vi "changeState.vi"(8 "error in (no error)":errorcluster, 10 "State":u16, 11 "Subnet in":refnum<class "Subnet.lvclass">) -> (0 "error out":errorcluster, 3 "Subnet out":refnum<class "Subnet.lvclass">)   [LabVIEW 2016, in "Subnet.lvclass"]
uses:
  Subnet.lvclass
  Subnet.lvclass/Subnet.ctl
  Common_RT_ILC/ILC/ILC.lvclass/ILC.ctl
  Common_RT_HPILC/HPILC/HPILC.lvclass
  D:/Code/Common_RT_ILC/ILC/ILC.lvclass
  Common_RT_MTILC/MTILC/MTILC.lvclass
  Common_RT_MDILC/MDILC/MDILC.lvclass
  Common_RT_MIILC/MIILC/MIILC.lvclass
  Common_RT_Modbus/IModbus/IModbus.lvclass
  Common_RT_ILC/ILC/ILC.lvclass
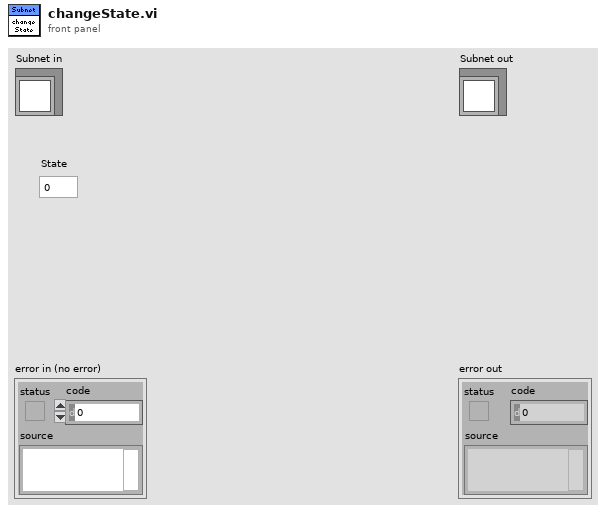
[diagram p1: front panel]
types:
  T1 = typedef "RTILC.lvlib/ILCData.ctl" = cluster{"Constants":T2, "Command":T3, "Telemetry":T5, "Responses":T6, "Timings":T8}
  T2 = typedef "RTILC.lvlib/ILCConstants.ctl" = cluster{"Subnet":u8, "Address":u8}
  T3 = typedef "RTILC.lvlib/ILCCommand.ctl" = cluster{"ILCMode":u16, "TemporaryAddress":u8, "ADCScanRate":T4, "ADCChannel":u8, "ADCOffset":sgl, "ADCSensitivity":sgl}
  T4 = typedef "RTILC.lvlib/ILCScanRates.ctl" = u8
  T5 = typedef "RTILC.lvlib/ILCTelemetry.ctl" = cluster{"UniqueID":u64, "FirmwareType":u8, "NetworkNodeType":u8, "ILCOption":u8, "NetworkNodeOption":u8, "MajorRevision":u8, "MinorRevision":u8, "FirmwareName":string, "ILCMode":u16, "MajorFault":bool, "MinorFault":bool, "FaultOverride":bool, "UniqueIDCRCMismatch":bool, "AppTypeNodeTypeMismatch":bool, "AppMissing":bool, "AppCRCMismatch":bool, "TEDSNotFound":bool, "TEDS1Mismatch":bool, "TEDS2Mismatch":bool, "WatchdogResetDetected":bool, "BrownoutDetected":bool, "EventTrapResetDetected":bool, "TemporaryAddress":u8, "ADCScanRate":T4, "DAC1":u16, "DAC2":u16, "DAC3":u16, "DAC4":u16, "MainADCCalibrationK":sgl[], "MainSensorOffset":sgl[], "MainSensorSensitivity":sgl[], "BackupADCCalibrationK":sgl[], "BackupSensorOffset":sgl[], "BackupSensorSensitivity":sgl[]}
  T6 = typedef "RTILC.lvlib/ILCResponses.ctl" = cluster{"ReportServerID":T7, "ReportServerStatus":T7, "ILCMode":T7, "SetTemporaryAddress":T7, "Reset":T7, "ADCScanRate":T7, "ADCOffsetSensitivity":T7, "ReadDAC":T7, "ReadCalibration":T7}
  T7 = typedef "RTModbus.lvlib/ExceptionCodes.ctl" = u16
  T8 = typedef "RTILC.lvlib/ILCTimings.ctl" = cluster{"ADCOffsetSensitivity":u32, "ADCScanRate":u32, "ILCMode":u32, "ReadCalibration":u32, "ReportServerID":u32, "ReportServerStatus":u32, "Reset":u32, "SetTemporaryAddress":u32}
  T9 = typedef "RTModbus.lvlib/TxFrame.ctl" = cluster{"Data":u8[], "WaitForTrigger":bool, "WaitForRx":u16, "TriggerIRQ":bool, "DelayMicroseconds":u16, "DelayMilliseconds":u16, "Timestamp":bool}
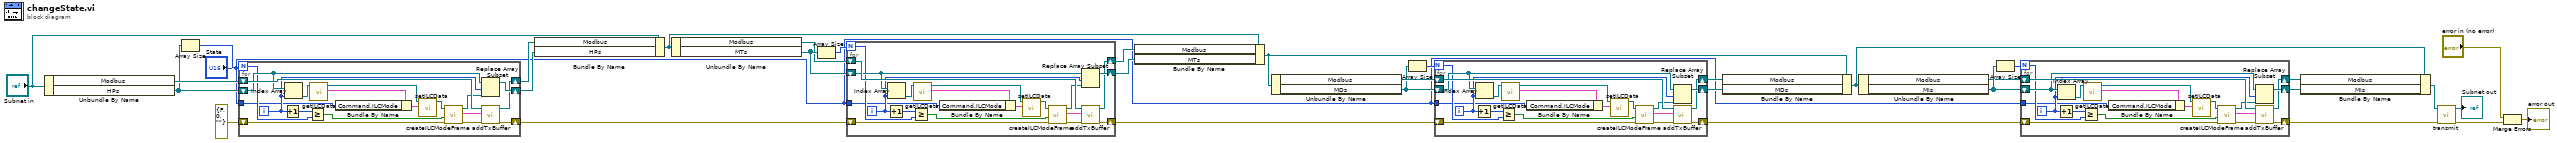
[diagram p0: block diagram]
diagram:
  n1 = Unbundle By Name("Subnet in") -> ("Modbus"=w35:refnum<class "IModbus.lvclass">, "HPs"=w34:refnum<class "HPILC.lvclass">[])
  n2 = Array Size(array=w34) -> (size(s)=w33:i32)
  n3 = for {
    N: w33 -> [w38]
    shift-right: [w44] -> w31
    shift-left: w35 -> [w49]
    shift-right: [w45] -> w30
    shift-left: w34 -> [w47]
    shift-right: [w42] -> w4
    shift-left: errorcluster {"status"=FALSE, "code"=0, "source"=""} ("error out") -> [w41]
    tunnel: "State" -> [w36]
    i -> [w40]
    n4 = Increment(x=w40) -> (x+1=w39:i32)
    n5 = Index Array(array=w47, index=w40) -> (element=w48:refnum<class "HPILC.lvclass">)
    n6 = Greater Or Equal?(x=w39, y=w38) -> (x >= y?=w37:bool)
    n7 = call "getILCData.vi"("ILC in"=w48) -> ("ILCData"=w53:T1, "ILC out"=w54:refnum<class "HPILC.lvclass">)  [unwired: 9 in]
    n8 = Bundle By Name(cluster=w53, "Command.ILCMode"=w36) -> (w52:T1)
    n9 = call "setILCData.vi"("ILCData"=w52, "ILC in"=w54) -> ("ILC out"=w51:refnum<class "HPILC.lvclass">)  [unwired: 9 in]
    n10 = call "createILCModeFrame.vi"("error in (no error)"=w41, "TriggerIRQ"=w37, "ILC in"=w51) -> ("error out"=w43:errorcluster, "TxFrame"=w50:T9, "ILC out"=w46:refnum<class "HPILC.lvclass">)  [unwired: 6 in]
    n11 = Replace Array Subset(array=w47, new element=w46, index=w40) -> (w45:refnum<class "HPILC.lvclass">[])
    n12 = call-dynamic "addTxBuffer.vi"("error in (no error)"=w43, "TxFrame"=w50, "IModbus in"=w49) -> ("error out"=w42:errorcluster, "IModbus out"=w44:refnum<class "IModbus.lvclass">)  [unwired: 7 in]
  }
  n13 = Bundle By Name(cluster="Subnet in", "Modbus"=w31, "HPs"=w30) -> (w19:refnum<class "Subnet.lvclass">)
  n14 = Unbundle By Name(w19) -> ("Modbus"=w20:refnum<class "IModbus.lvclass">, "MTs"=w21:refnum<class "MTILC.lvclass">[])
  n15 = Array Size(array=w21) -> (size(s)=w22:i32)
  n16 = for {
    N: w22 -> [w57]
    shift-right: [w63] -> w23
    shift-left: w20 -> [w68]
    shift-right: [w64] -> w24
    shift-left: w21 -> [w66]
    shift-right: [w61] -> w5
    shift-left: w4 -> [w60]
    tunnel: "State" -> [w55]
    i -> [w59]
    n17 = Increment(x=w59) -> (x+1=w58:i32)
    n18 = Index Array(array=w66, index=w59) -> (element=w67:refnum<class "MTILC.lvclass">)
    n19 = Greater Or Equal?(x=w58, y=w57) -> (x >= y?=w56:bool)
    n20 = call "getILCData.vi"("ILC in"=w67) -> ("ILCData"=w72:T1, "ILC out"=w73:refnum<class "MTILC.lvclass">)  [unwired: 9 in]
    n21 = Bundle By Name(cluster=w72, "Command.ILCMode"=w55) -> (w71:T1)
    n22 = call "setILCData.vi"("ILCData"=w71, "ILC in"=w73) -> ("ILC out"=w70:refnum<class "MTILC.lvclass">)  [unwired: 9 in]
    n23 = call "createILCModeFrame.vi"("error in (no error)"=w60, "TriggerIRQ"=w56, "ILC in"=w70) -> ("error out"=w62:errorcluster, "TxFrame"=w69:T9, "ILC out"=w65:refnum<class "MTILC.lvclass">)  [unwired: 6 in]
    n24 = Replace Array Subset(array=w66, new element=w65, index=w59) -> (w64:refnum<class "MTILC.lvclass">[])
    n25 = call-dynamic "addTxBuffer.vi"("error in (no error)"=w62, "TxFrame"=w69, "IModbus in"=w68) -> ("error out"=w61:errorcluster, "IModbus out"=w63:refnum<class "IModbus.lvclass">)  [unwired: 7 in]
  }
  n26 = Bundle By Name(cluster=w19, "Modbus"=w23, "MTs"=w24) -> (w13:refnum<class "Subnet.lvclass">)
  n27 = Unbundle By Name(w13) -> ("Modbus"=w18:refnum<class "IModbus.lvclass">, "MDs"=w17:refnum<class "MDILC.lvclass">[])
  n28 = Array Size(array=w17) -> (size(s)=w16:i32)
  n29 = for {
    N: w16 -> [w76]
    shift-right: [w82] -> w15
    shift-left: w18 -> [w87]
    shift-right: [w83] -> w14
    shift-left: w17 -> [w85]
    shift-right: [w80] -> w6
    shift-left: w5 -> [w79]
    tunnel: "State" -> [w74]
    i -> [w78]
    n30 = Increment(x=w78) -> (x+1=w77:i32)
    n31 = Index Array(array=w85, index=w78) -> (element=w86:refnum<class "MDILC.lvclass">)
    n32 = Greater Or Equal?(x=w77, y=w76) -> (x >= y?=w75:bool)
    n33 = call "getILCData.vi"("ILC in"=w86) -> ("ILCData"=w91:T1, "ILC out"=w92:refnum<class "MDILC.lvclass">)  [unwired: 9 in]
    n34 = Bundle By Name(cluster=w91, "Command.ILCMode"=w74) -> (w90:T1)
    n35 = call "setILCData.vi"("ILCData"=w90, "ILC in"=w92) -> ("ILC out"=w89:refnum<class "MDILC.lvclass">)  [unwired: 9 in]
    n36 = call "createILCModeFrame.vi"("error in (no error)"=w79, "TriggerIRQ"=w75, "ILC in"=w89) -> ("error out"=w81:errorcluster, "TxFrame"=w88:T9, "ILC out"=w84:refnum<class "MDILC.lvclass">)  [unwired: 6 in]
    n37 = Replace Array Subset(array=w85, new element=w84, index=w78) -> (w83:refnum<class "MDILC.lvclass">[])
    n38 = call-dynamic "addTxBuffer.vi"("error in (no error)"=w81, "TxFrame"=w88, "IModbus in"=w87) -> ("error out"=w80:errorcluster, "IModbus out"=w82:refnum<class "IModbus.lvclass">)  [unwired: 7 in]
  }
  n39 = Bundle By Name(cluster=w13, "Modbus"=w15, "MDs"=w14) -> (w7:refnum<class "Subnet.lvclass">)
  n40 = Unbundle By Name(w7) -> ("Modbus"=w8:refnum<class "IModbus.lvclass">, "MIs"=w9:refnum<class "MIILC.lvclass">[])
  n41 = Array Size(array=w9) -> (size(s)=w10:i32)
  n42 = for {
    N: w10 -> [w95]
    shift-right: [w101] -> w11
    shift-left: w8 -> [w106]
    shift-right: [w102] -> w12
    shift-left: w9 -> [w104]
    shift-right: [w99] -> w3
    shift-left: w6 -> [w98]
    tunnel: "State" -> [w93]
    i -> [w97]
    n43 = Increment(x=w97) -> (x+1=w96:i32)
    n44 = Index Array(array=w104, index=w97) -> (element=w105:refnum<class "MIILC.lvclass">)
    n45 = Greater Or Equal?(x=w96, y=w95) -> (x >= y?=w94:bool)
    n46 = call "getILCData.vi"("ILC in"=w105) -> ("ILCData"=w110:T1, "ILC out"=w111:refnum<class "MIILC.lvclass">)  [unwired: 9 in]
    n47 = Bundle By Name(cluster=w110, "Command.ILCMode"=w93) -> (w109:T1)
    n48 = call "setILCData.vi"("ILCData"=w109, "ILC in"=w111) -> ("ILC out"=w108:refnum<class "MIILC.lvclass">)  [unwired: 9 in]
    n49 = call "createILCModeFrame.vi"("error in (no error)"=w98, "TriggerIRQ"=w94, "ILC in"=w108) -> ("error out"=w100:errorcluster, "TxFrame"=w107:T9, "ILC out"=w103:refnum<class "MIILC.lvclass">)  [unwired: 6 in]
    n50 = Replace Array Subset(array=w104, new element=w103, index=w97) -> (w102:refnum<class "MIILC.lvclass">[])
    n51 = call-dynamic "addTxBuffer.vi"("error in (no error)"=w100, "TxFrame"=w107, "IModbus in"=w106) -> ("error out"=w99:errorcluster, "IModbus out"=w101:refnum<class "IModbus.lvclass">)  [unwired: 7 in]
  }
  n52 = Bundle By Name(cluster=w7, "Modbus"=w11, "MIs"=w12) -> (w2:refnum<class "Subnet.lvclass">)
  n53 = call "transmit.vi"("error in (no error)"=w3, "Subnet in"=w2) -> ("error out"=w26:errorcluster, "Subnet out"=→"Subnet out":refnum<class "Subnet.lvclass">)  [unwired: 8 in]
  n54 = Merge Errors("error in (no error)", w26) -> (→"error out":errorcluster)
